vi "FTW-Actor-HandleEvents.vi"(0 "FTW-ActorInstance In":refnum<class "FTW-ActorInstance.lvclass">, 5 "FTW Incoming Request In":refnum<class "FTW-Message-IncomingRequest.lvclass">, 11 "error in":errorcluster) -> (4 "FTW-ActorInstance Out":refnum<class "FTW-ActorInstance.lvclass">, 6 "FTW Incoming Request":refnum<class "FTW-Message-IncomingRequest.lvclass">, 15 "error out":errorcluster)   [LabVIEW 2015, in "FTW-ActorInstance.lvclass"]
uses:
  FTW-ActorInstance.lvclass
  Message/Request/FTW-Message-IncomingRequest.lvclass
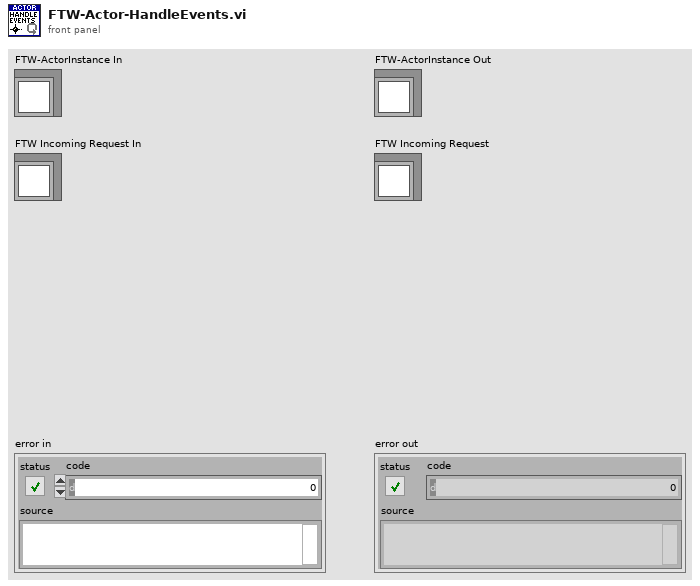
[diagram p1: front panel]
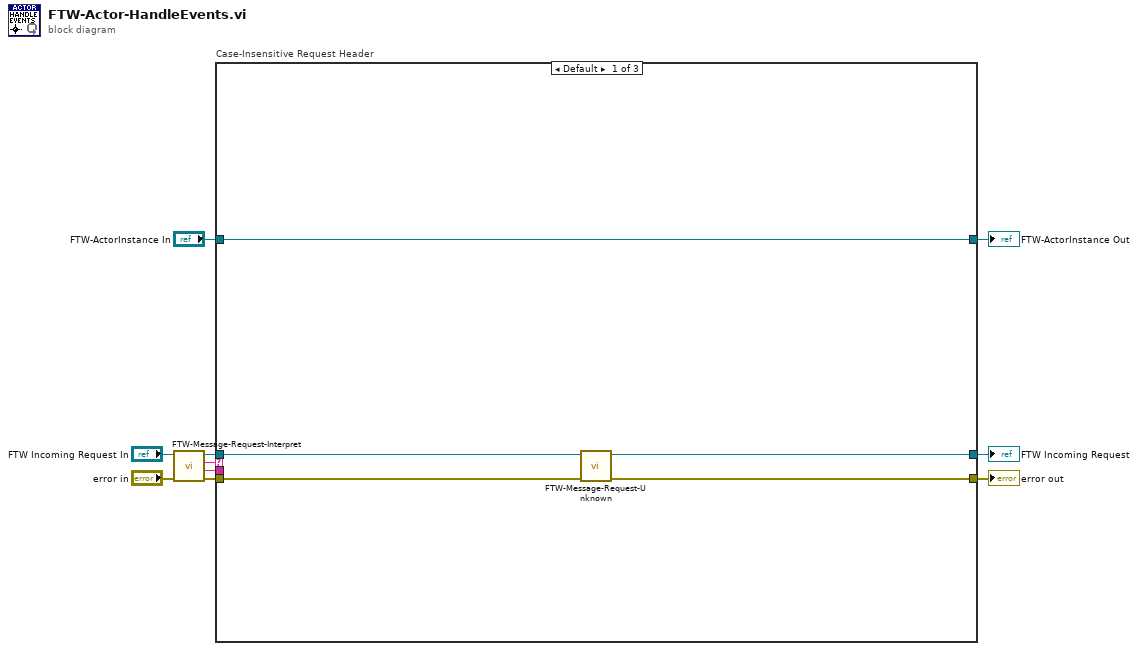
[diagram p0: block diagram]
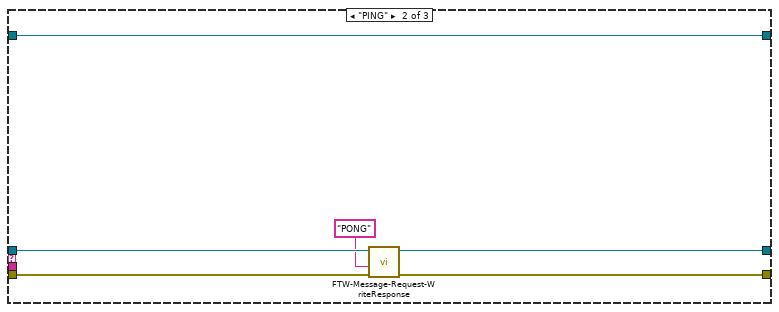
[diagram p2: hidden frame]
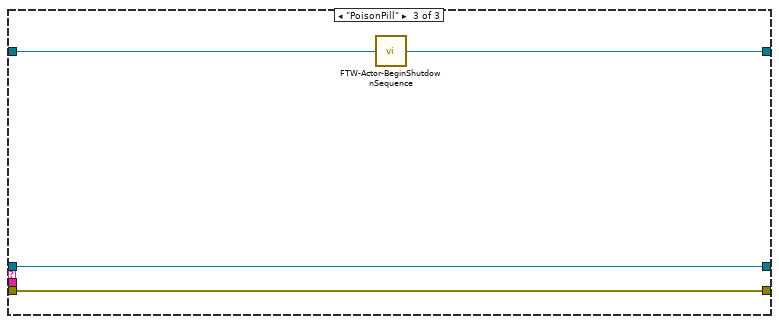
[diagram p3: hidden frame]
diagram:
  n1 = call "FTW-Message-Request-Interpret.vi"("error in"="error in", "FTW Incoming Request"="FTW Incoming Request In") -> ("error out"=w10:errorcluster, "Request Body"=w8:string, "Request Header"=w9:string, "FTW Incoming Request out"=w7:refnum<class "FTW-Message-IncomingRequest.lvclass">)  [unwired: 6 in]
  n2 = case "Case-Insensitive Request Header" shown="Default" w9 {
    tunnel: [w13 w19 w24] -> w1
    tunnel: w10 -> [w14 w20 w24]
    tunnel: [w15 w18 w25] -> w3
    tunnel: "FTW-ActorInstance In" -> [w15 w18 w23]
    tunnel: w7 -> [w12 w21 w22]
    tunnel: [w11 w17 w22] -> w2
    tunnel: w8 -> [_ _ _]
    frame Default {
      n3 = call "FTW-Message-Request-Unknown.vi"("error in"=w14, "FTW Incoming Request"=w12) -> ("error out"=w13:errorcluster, "FTW Incoming Request Out"=w11:refnum<class "FTW-Message-IncomingRequest.lvclass">)  [unwired: 8 in]
    }
    frame "PING" {
      n4 = call "FTW-Message-Request-WriteResponse.vi"("error in"=w20, "Response Body"="PONG" ("Response Header"), "FTW Incoming Request"=w21) -> ("error out"=w19:errorcluster, "FTW Incoming Request out"=w17:refnum<class "FTW-Message-IncomingRequest.lvclass">)  [unwired: 7 in]
    }
    frame "PoisonPill" {
      n5 = call "FTW-Actor-BeginShutdownSequence.vi"("FTW Actor Instance"=w23) -> ("FTW Actor Instance out"=w25:refnum<class "FTW-ActorInstance.lvclass">)  [unwired: 3 in]
    }
  }
  "FTW-ActorInstance Out" <- w3
  "error out" <- w1
  "FTW Incoming Request" <- w2
